vi "Module Name--constant.vi"() -> (3 "Module Name":string)   [LabVIEW 2022 SP3, in "Dummy.lvlib"]
doc: "Return the name of the module that owns this VI. \n____\nHAMPEL SOFTWARE ENGINEERING v2.6.0 (2023-12-19 10:54)"
uses:
  Dummy.lvlib
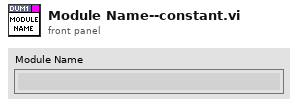
[diagram p1: front panel]
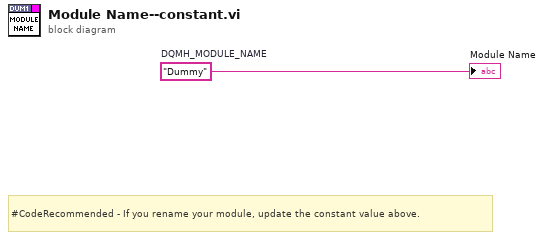
[diagram p0: block diagram]
diagram:
  w1 = "Dummy"  # DQMH_MODULE_NAME
  # "#CodeRecommended - If you rename your module, update the constant value above."
  "Module Name" <- w1
